vi "Generate FilenameRU.vi"(8 "error in":errorcluster, 11 "Log in":refnum<class "Log.lvclass">) -> (0 "error out":errorcluster, 3 "Log out":refnum<class "Log.lvclass">)   [LabVIEW 2017, in "Report_lib.lvlib" / "Log.lvclass"]
doc: "This SubVI generate filename based on\ncurrent data by polimorphic GenFilename.vi"
uses:
  Log.lvclass
  Log.lvclass/Log.ctl
  <vilib>/regexp/Match Regular Expression.xnode
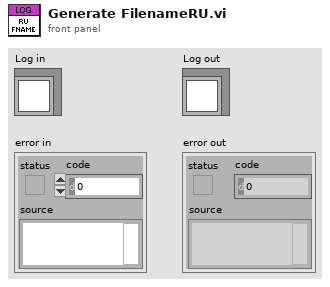
[diagram p1: front panel]
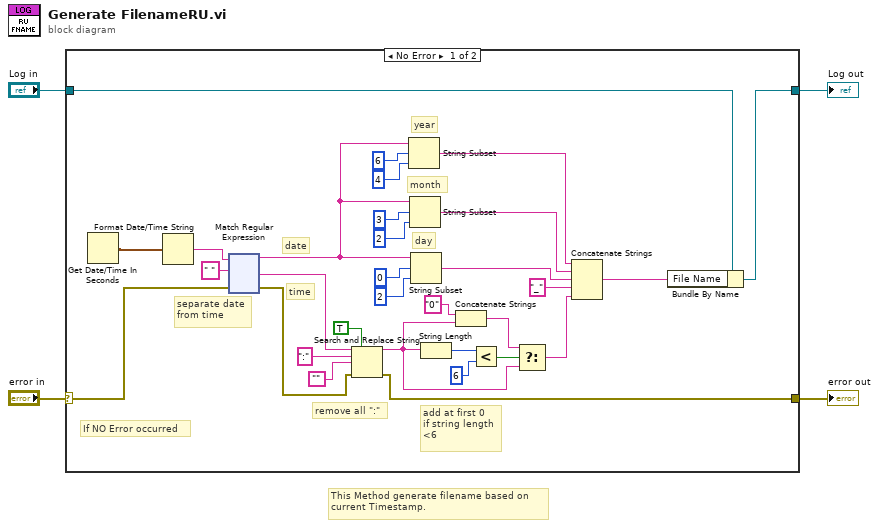
[diagram p0: block diagram]
diagram:
  # "This Method generate filename based on\ncurrent Timestamp."
  n1 = case shown="No Error" "error in" {
    selector: "error in" -> [w32 w151]
    tunnel: [w30 w151] -> w3
    tunnel: [w34 w150] -> w1
    tunnel: "Log in" -> [w35 w150]
    frame No Error {
      # "add at first 0\nif string length\n<6"
      # "remove all \":\""
      # "separate date \nfrom time"
      # "time"
      # "date"
      # "day"
      # "month"
      # "year"
      # "If NO Error occurred"
      n2 = Get Date/Time In Seconds() -> (seconds since 1Jan1904=w33:timestamp)
      n3 = Format Date/Time String(seconds (now)=w33) -> (date/time string=w29:string)  [unwired: 2 in]
      n4 = xnode "Match Regular Expression"("input string"=w29, "regular expression"=" ", "error in"=w32) -> ("before match"=w17:string, "after match"=w19:string, "error out"=w9:errorcluster)  [unwired: 3 in, 2 out]
      n5 = Search and Replace String(replace all?=TRUE ("replace all? (F)"), input string=w19, search string=":", replace string="", error in=w9) -> (result string=w24:string, error out=w30:errorcluster)  [unwired: 3 in, 2 out]
      n6 = String Subset(string=w17, offset (0)=6, length (rest)=4 ("length (rest)")) -> (substring=w7:string)
      n7 = String Subset(string=w17, offset (0)=3, length (rest)=2 ("length (rest)")) -> (substring=w6:string)
      n8 = String Subset(string=w17, offset (0)=0, length (rest)=2 ("length (rest)")) -> (substring=w5:string)
      n9 = String Length(string=w24) -> (length=w21:i32)
      n10 = Concatenate Strings("0" ("string"), w24) -> (w26:string)
      n11 = Less?(x=w21, y=6) -> (x < y?=w23:bool)
      n12 = Select(t=w26, s=w23, f=w24) -> (s? t:f=w28:string)
      n13 = Concatenate Strings(w7, w6, w5, "_" ("string"), w28) -> (w31:string)
      n14 = Bundle By Name(cluster=w35, "File Name"=w31) -> (w34:refnum<class "Log.lvclass">)
    }
    frame Error {
    }
  }
  "error out" <- w3
  "Log out" <- w1
